vi "TDMS File Viewer.vi"() -> ()   [LabVIEW 2015]
panel:
  in  "file path":path
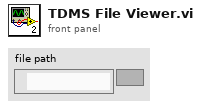
[diagram p1: front panel]
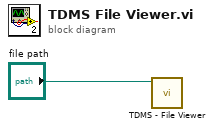
[diagram p0: block diagram]
diagram:
  n1 = call <vilib>:"TDMS - File Viewer.vi"("file path"="file path") -> ()  [unwired: 5 in, 2 out]
